vi "DHE_template2keys.vi"(8 "error in (no error)":errorcluster, 9 "HdrInfo In":string[][](array[string]), 10 "Action":T1(ring), 11 "file":path=path "/home/arcconfig/DHE_INFO.tpl") -> (0 "error out":errorcluster, 2 "number of keywords found":i32, 3 "HdrInfo":string[][](table))   [LabVIEW 2016]
doc: "This VI reads the configuration file searching for the \"infofile\" keyword. Then, it goes and reads the specified file, which should be a template for the TCS info format"
uses:
  private/vis/DHE_TP_action.ctl
  <vilib>/Utility/config.llb/Read Key (String).vi
  <vilib>/Utility/config.llb/NI_LVConfig.lvlib
panel:
  in  "default hdr file":path=path "/home/arcconfig/DHE_INFO.tpl"
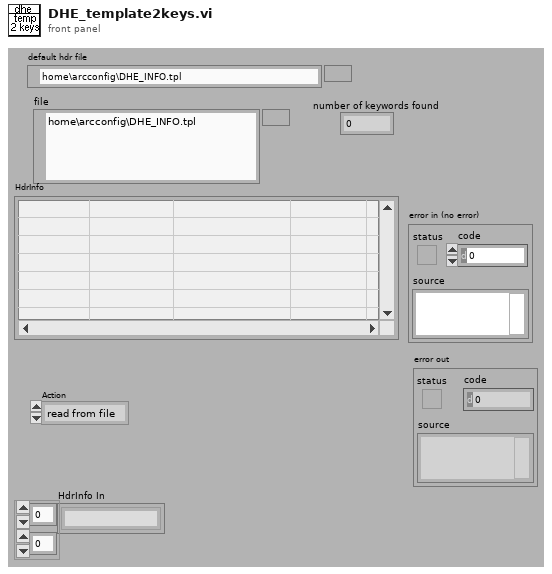
[diagram p1: front panel]
types:
  T1 = enum16{"read from file", "clear", "get all", "set all"}
  T2 = typedef "NI_LVConfig.lvlib/Config Data RefNum.ctl" = refnum<k1>
  T3 = typedef "DHE_TP_action.ctl" = enum16{"READ FROM FILE", "GET ALL", "FIND BY NAME", "FIND BY TYPE", "SET VALUE", "CLEAN", "CHANGE", "GET EXPUPDATE"}
  T4 = typedef "DHE_TP.ctl" = cluster{"name":string, "type":string, "R_algor":string[], "board":string, "memory":string, "address":i32, "value":string, "Limits":T5, "unit":string, "params":string, "permissions":string, "W_algor":string[], "description":string, "err_count":i32, "max_err":i32, "read":bool, "lowrej":dbl, "hirej":dbl, "expupd":bool}
  T5 = typedef "DHE_TPLimits.ctl" = cluster{"upper":dbl, "Lower":dbl, "InRange":bool, "nominal":dbl}
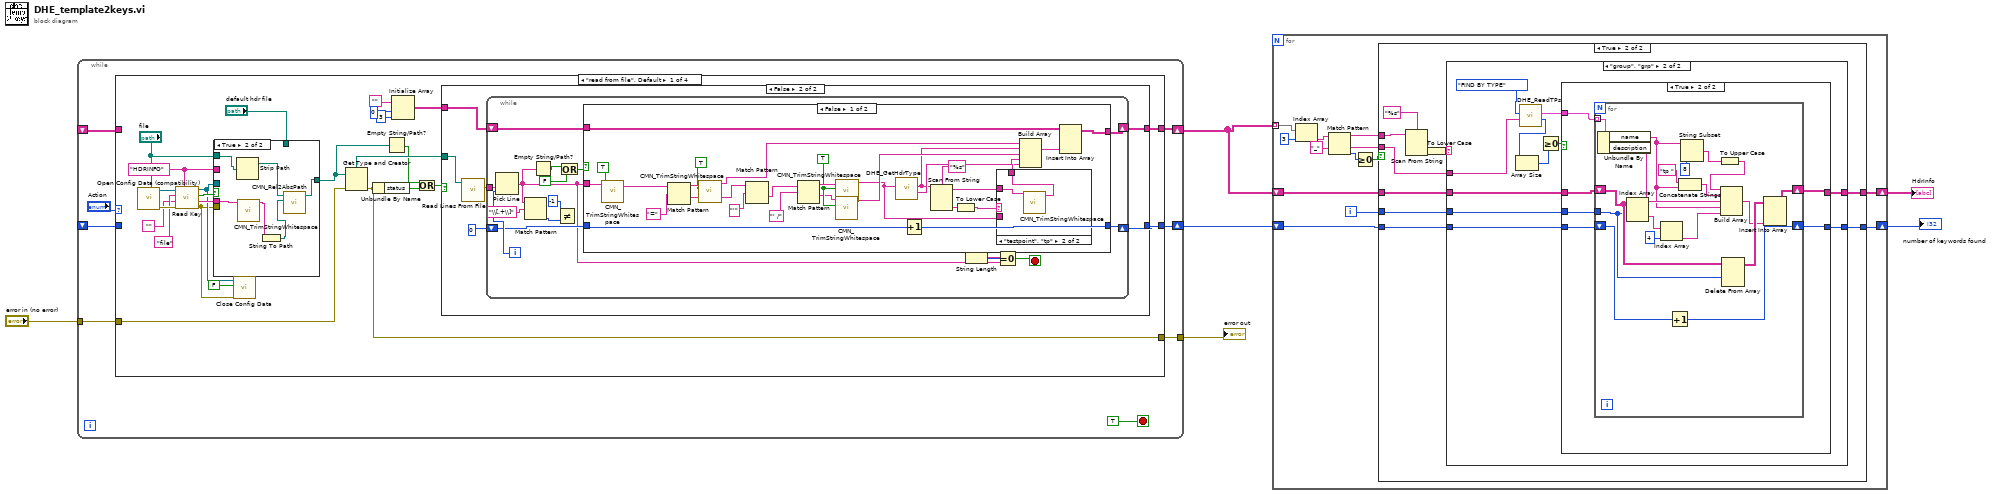
[diagram p0: block diagram]
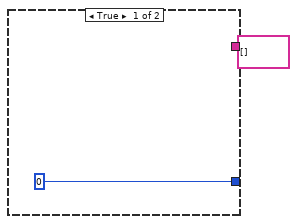
[diagram p6: hidden frame]
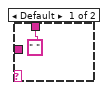
[diagram p7: hidden frame]
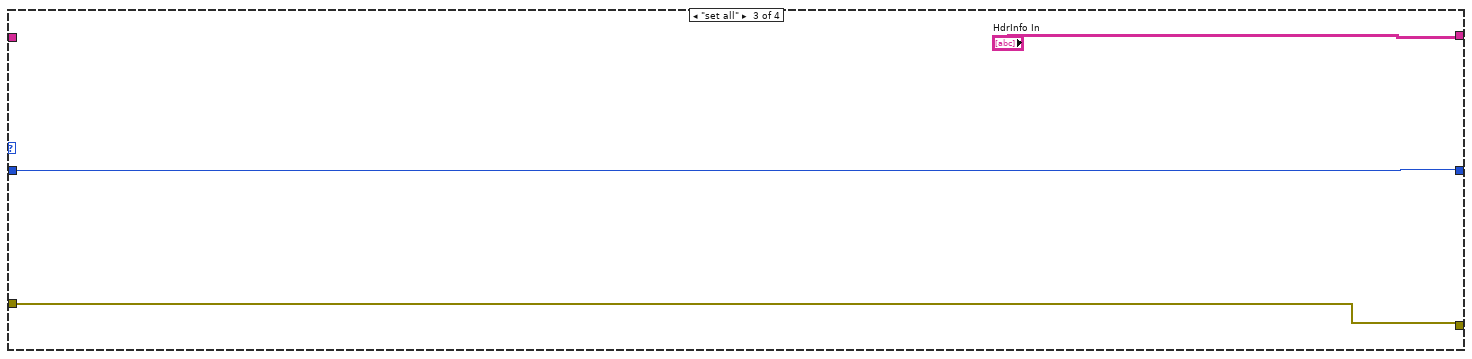
[diagram p10: hidden frame]
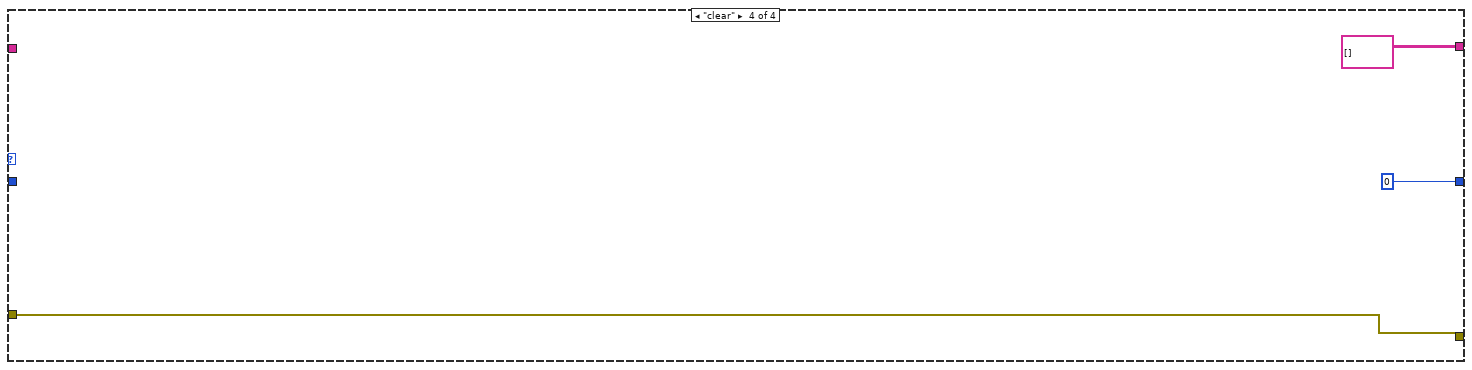
[diagram p11: hidden frame]
diagram:
  n1 = while {
    shift-right: [w13] -> w4
    shift-left: _ -> [w11]
    tunnel: [w10] -> w6
    shift-right: [w9] -> w2
    shift-left: _ -> [w8]
    tunnel: "error in (no error)" -> [w7]
    stop <- TRUE stop-if-true
    n2 = case shown="\"read from file\", Default" "Action" {
      tunnel: [w24 w104 "HdrInfo In" string[][] []] -> w13
      tunnel: w11 -> [_ w104 _ _]
      tunnel: [w23 w102 w106 w108] -> w10
      tunnel: [w22 w103 w107 0] -> w9
      tunnel: w8 -> [_ w103 w107 _]
      tunnel: w7 -> [w21 w102 w106 w108]
      frame "read from file", Default {
        w28 = "HDRINFO" ("section")
        n3 = call <vilib>:"Open Config Data (compatibility).vi"("configuration file path"="file") -> ("error out"=w33:errorcluster, "refnum"=w34:T2)  [unwired: 8 in, 1 out]
        n4 = call-poly <vilib>:"Read Key.vi"("section"=w28, "error in (no error)"=w33, "default value"="", "key"="file", "refnum"=w34) -> ("error out"=w25:errorcluster, "value"=w29:string, "found?"=w30:bool, "refnum out"=w26:T2)  [unwired: 1 in, 2 out]
        n5 = case shown="True" w30 {
          tunnel: w29 -> [_ w45]
          tunnel: [w39 w42] -> w18
          tunnel: w26 -> [_ _]
          tunnel: w25 -> [_ _]
          tunnel: w28 -> [_ _]
          tunnel: "default hdr file" -> [w39 _]
          tunnel: "file" -> [_ w41]
          frame False {
          }
          frame True {
            n6 = Strip Path(path=w41) -> (stripped path=w40:path)  [unwired: 1 out]
            n7 = call "CMN_TrimStringWhitespace.vi"("string"=w45) -> ("trimmed string"=w44:string)  [unwired: 1 in, 8 out]
            n8 = String To Path(string=w44) -> (path=w43:path)
            n9 = call "CMN_Rel2AbsPath.vi"("test path"=w43, "absolute path"=w40) -> ("output path"=w42:path)  [unwired: 1 in, 8 out]
          }
        }
        n10 = call <vilib>:"Close Config Data.vi"("error in (no error)"=w25, "write file if changed (T)"=FALSE ("write configuration file? (T)"), "refnum"=w26) -> ()  [unwired: 9 out]
        n11 = Get Type and Creator(4:w21, 7:w18) -> (0:w23:errorcluster)  [unwired: 3 out]
        n12 = Unbundle By Name(w23) -> ("status"=w19:bool)
        n13 = Empty String/Path?(string/path=w18) -> (empty?=w17:bool)
        n14 = Initialize Array("", 0, 3 ("dimension size")) -> (w36:string[][])
        n15 = Or(x=w17, y=w19) -> (x .or. y?=w16:bool)
        n16 = case shown="False" w16 {
          tunnel: w18 -> [_ w52]
          tunnel: [0 w49] -> w22
          tunnel: [string[][] [] w48] -> w24
          tunnel: w36 -> [_ w51]
          frame True {
          }
          frame False {
            n17 = call <vilib>:"Read Lines From File.vi"("file path (dialog if empty)"=w52) -> ("line string"=w53:string)  [unwired: 1 in, 7 out]
            n18 = while {
              shift-left: 0 -> [w58]
              shift-right: [w60] -> w49
              shift-left: w51 -> [w65]
              shift-right: [w64] -> w48
              tunnel: w53 -> [w68]
              i -> [w59]
              stop <- w66 stop-if-true
              n19 = Pick Line(multi-line string=w68, line index=w59) -> (output string=w56:string)  [unwired: 1 out]
              n20 = Match Pattern(string=w56, regular expression="\\[.+\\]") -> (offset past match=w62:i32)  [unwired: 4 out]
              n21 = Empty String/Path?(string/path=w56) -> (empty?=w57:bool)
              n22 = Not Equal?(x=-1, y=w62) -> ()  [unwired: 1 out]
              n23 = Or(x=w57, y=FALSE) -> (x .or. y?=w55:bool)
              n24 = case shown="False" w55 {
                tunnel: w58 -> [w81 w100]
                tunnel: w65 -> [w85 w101]
                tunnel: [w84 w101] -> w64
                tunnel: [w80 w100] -> w60
                tunnel: w56 -> [w79 _]
                frame False {
                  w88 = TRUE ("Both Ends?(F)")
                  n25 = call "CMN_TrimStringWhitespace.vi"("Both Ends?(T)"=TRUE ("Both Ends?(F)"), "string"=w79) -> ("trimmed string"=w78:string)  [unwired: 8 out]
                  n26 = Match Pattern(string=w78, regular expression="=") -> (before substring=w95:string, after substring=w94:string)  [unwired: 3 out]
                  n27 = call "CMN_TrimStringWhitespace.vi"("Both Ends?(T)"=TRUE ("Both Ends?(F)"), "string"=w95) -> ("trimmed string"=w82:string)  [unwired: 8 out]
                  n28 = Match Pattern(string=w94, regular expression="'") -> (after substring=w92:string)  [unwired: 4 out]
                  n29 = Match Pattern(string=w92, regular expression="' /") -> (before substring=w90:string, after substring=w87:string)  [unwired: 3 out]
                  n30 = call "CMN_TrimStringWhitespace.vi"("Both Ends?(T)"=w88, "string"=w87) -> ("trimmed string"=w74:string)  [unwired: 8 out]
                  n31 = call "CMN_TrimStringWhitespace.vi"("Both Ends?(T)"=w88, "string"=w90) -> ("trimmed string"=w71:string)  [unwired: 8 out]
                  n32 = call "DHE_GetHdrType.vi"("keyval"=w71) -> ("type"=w70:string, "keyval out"=w69:string)  [unwired: 9 out]
                  n33 = Increment(x=w81) -> (x+1=w80:i32)
                  n34 = Scan From String(format string="%s", input string=w69) -> (remaining string=w72:string, output 1=w76:string)  [unwired: 2 in, 3 out]
                  n35 = To Lower Case(string=w76) -> (all lower case string=w75:string)
                  n36 = case shown="\"testpoint\", \"tp\"" w75 {
                    tunnel: [" " w98] -> w73
                    tunnel: w72 -> [_ w99]
                    tunnel: w71 -> [_ _]
                    frame Default {
                    }
                    frame "testpoint", "tp" {
                      n37 = call "CMN_TrimStringWhitespace.vi"("string"=w99) -> ("trimmed string"=w98:string)  [unwired: 1 in, 8 out]
                    }
                  }
                  n38 = Build Array(w82, w69, w74, w73, w70) -> (w86:string[])
                  n39 = Insert Into Array(array=w85, new element=w86) -> (w84:string[][])  [unwired: 2 in]
                }
                frame True {
                }
              }
              n40 = String Length(string=w56) -> (length=w67:i32)
              n41 = Equal To 0?(x=w67) -> (x = 0?=w66:bool)
            }
          }
        }
      }
      frame "get all" {
      }
      frame "set all" {
      }
      frame "clear" {
      }
    }
  }
  "error out" <- w6
  n42 = for {
    tunnel: w4 -> [w123] mode=indexing
    shift-right: [w114] -> w3
    shift-left: w4 -> [w115]
    shift-right: [w112] -> w1
    shift-left: w2 -> [w113]
    i -> [w111]
    n43 = Index Array(array=w123, index=3) -> (element=w121:string)
    n44 = Match Pattern(string=w121, regular expression="_") -> (before substring=w117:string, after substring=w116:string, offset past match=w119:i32)  [unwired: 2 out]
    n45 = Greater Or Equal To 0?(x=w119) -> (x >= 0?=w118:bool)
    n46 = case shown="True" w118 {
      tunnel: w117 -> [_ w135]
      tunnel: w116 -> [_ w126]
      tunnel: w115 -> [w125 w131]
      tunnel: [w125 w130] -> w114
      tunnel: w113 -> [w124 w129]
      tunnel: [w124 w128] -> w112
      tunnel: w111 -> [_ w127]
      frame False {
      }
      frame True {
        n47 = Scan From String(format string="%s", input string=w135) -> (output 1=w133:string)  [unwired: 2 in, 4 out]
        n48 = To Lower Case(string=w133) -> (all lower case string=w132:string)
        n49 = case shown="\"group\", \"grp\"" w132 {
          tunnel: w131 -> [w137 w147]
          tunnel: [w137 w146] -> w130
          tunnel: w129 -> [w136 w145]
          tunnel: [w136 w144] -> w128
          tunnel: w127 -> [_ w142]
          tunnel: w126 -> [_ w141]
          frame Default {
          }
          frame "group", "grp" {
            n50 = call "DHE_ReadTPs.vi"("argument"=w141, "action"=DHE_TP_action."FIND BY TYPE") -> ("index"=w139:i32[], "TPs"=w143:T4[])  [unwired: 5 in, 3 out]
            n51 = Array Size(array=w139) -> (size(s)=w138:i32)
            n52 = Greater Or Equal To 0?(x=w138) -> (x >= 0?=w148:bool)
            n53 = case shown="True" w148 {
              tunnel: w147 -> [w150 w155]
              tunnel: [w150 w153] -> w146
              tunnel: w145 -> [w149 w154]
              tunnel: [w149 w152] -> w144
              tunnel: w143 -> [_ w156]
              tunnel: w142 -> [_ w151]
              frame False {
              }
              frame True {
                n54 = for {
                  tunnel: w156 -> [w174] mode=indexing
                  shift-right: [w160] -> w153
                  shift-left: w155 -> [w164]
                  shift-right: [w165] -> w152
                  shift-left: w154 -> [w166]
                  tunnel: w151 -> [w163]
                  n55 = Unbundle By Name(w174) -> ("name"=w157:string, "description"=w170:string)
                  n56 = Index Array(array=w164, index (row)=w163) -> (element=w169:string[])  [unwired: 1 in]
                  n57 = Index Array(array=w169, index=4) -> (element=w167:string)
                  n58 = Increment(x=w166) -> (x+1=w165:i32)
                  n59 = Concatenate Strings("tp " ("string"), w157) -> (w158:string)
                  n60 = String Subset(string=w157, length (rest)=8 ("length (rest)")) -> (substring=w172:string)  [unwired: 1 out]
                  n61 = To Upper Case(1:w172) -> (0:w171:string)
                  n62 = Build Array(w171, w158, w170, w157, w167) -> (w161:string[])
                  n63 = Delete From Array(array=w164, index (row)=w163) -> (array with subset deleted=w162:string[][])  [unwired: 2 in, 1 out]
                  n64 = Insert Into Array(array=w162, new element=w161) -> (w160:string[][])  [unwired: 2 in]
                }
              }
            }
          }
        }
      }
    }
  }
  "number of keywords found" <- w1
  "HdrInfo" <- w3
